vi "test5-AsyncMessageWithReply.vi"(8 "error in (no error)":errorcluster, 11 "TestCase in":refnum<class "testcase-CSMMessage.lvclass">) -> (0 "error out":errorcluster, 3 "TestCase out":refnum<class "testcase-CSMMessage.lvclass">)   [LabVIEW 2017, in "testcase-CSMMessage.lvclass"]
uses:
  testcase-CSMMessage.lvclass
  7412589e-de49-4983-aece-358686b48526.vi
  src/user.lib/_NEVSTOP/Communicable State Machine(CSM)/AdvanceAPI/CSM - Make String Arguments Safe.vi
  src/user.lib/_NEVSTOP/Communicable State Machine(CSM)/AdvanceAPI/CSM - Keywords.vi
  <vilib>/addons/_JKI Toolkits/VI Tester/TestCase.llb/TestCase.lvclass
  src/user.lib/_NEVSTOP/Communicable State Machine(CSM)/Communicable State Machine.lvlib
  C:/Program Files (x86)/National Instruments/LabVIEW 2017/vi.lib/addons/_JKI Toolkits/VI Tester/TestCase.llb/TestCase.lvclass
panel:
  out "Loop count":i32
  out "debug message":string
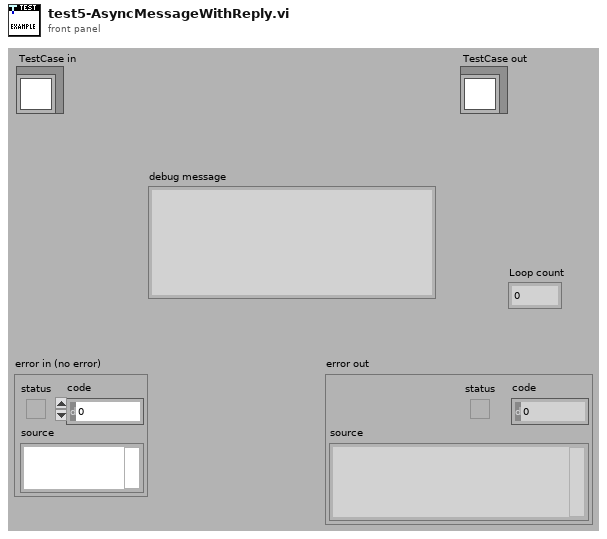
[diagram p1: front panel]
types:
  T1 = cluster{"Arguments":string, "Response":string, "error":errorcluster}
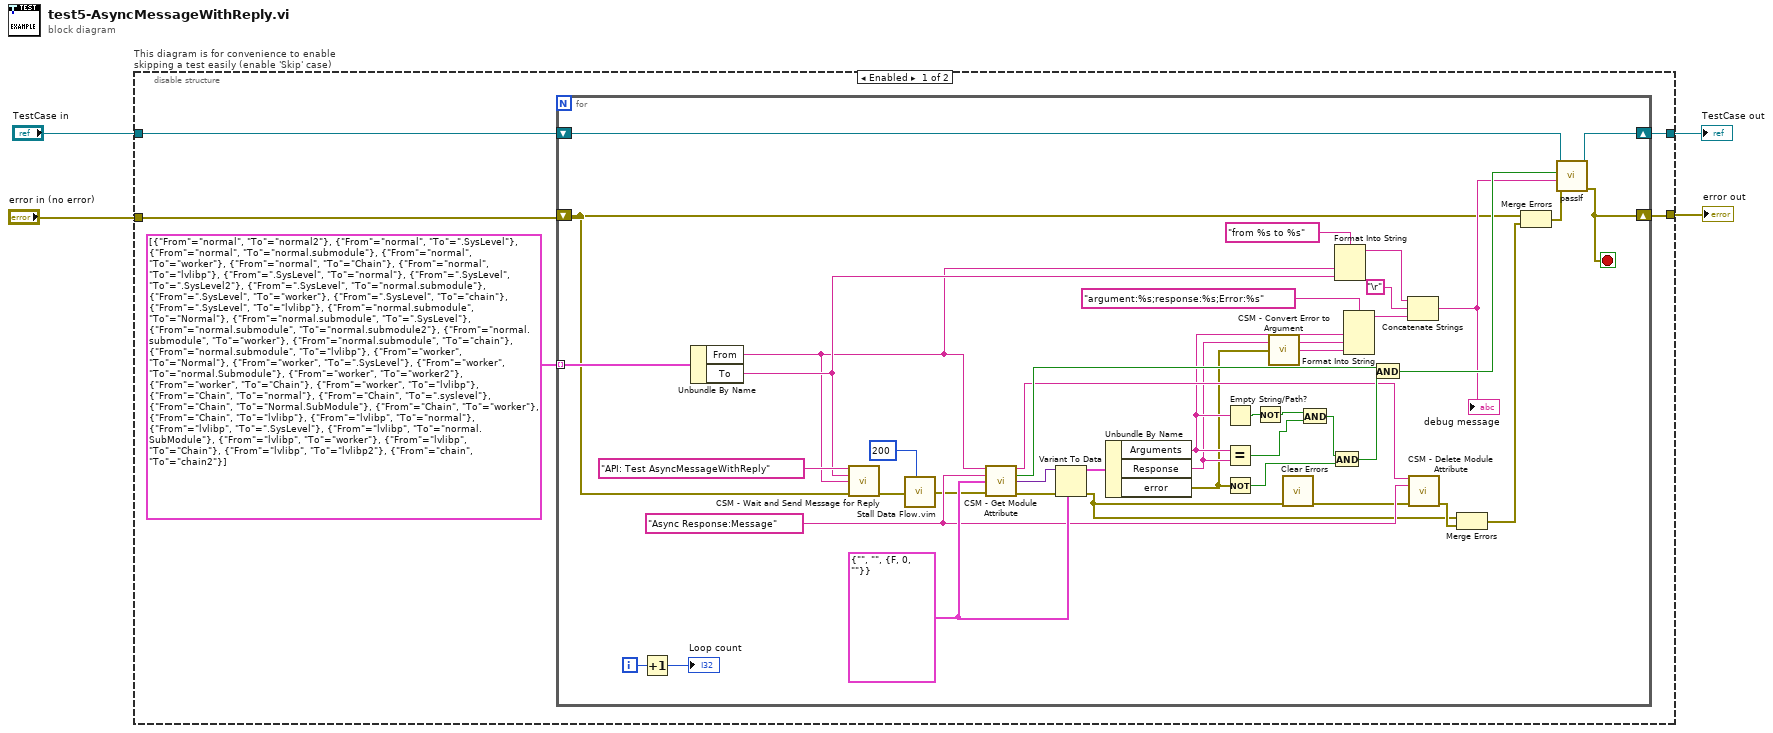
[diagram p0: block diagram]
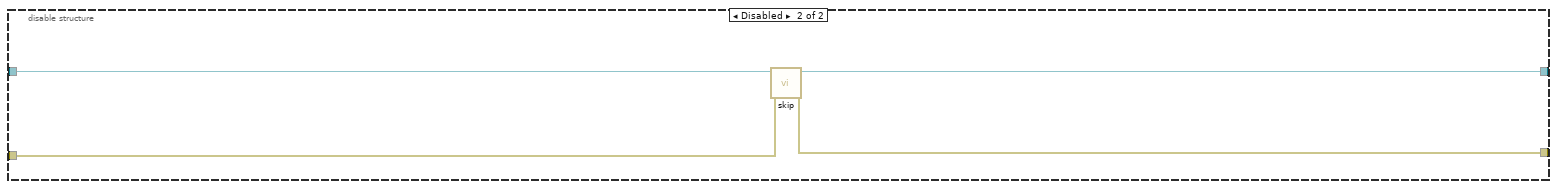
[diagram p2: hidden frame]
diagram:
  n1 = disable-structure "This diagram is for convenience to enable skipping a test easily (enable 'Skip' case)" shown="Enabled" {
    disable-tunnel: "TestCase in" -> [w9 w55]
    disable-tunnel: [w8 w53] -> w1
    disable-tunnel: [w5 w54] -> w3
    disable-tunnel: "error in (no error)" -> [w7 w52]
    frame Enabled {
      n2 = for {
        tunnel: cluster{"From":string, "To":string}[] [{"From"="normal", "To"="normal2"}, {"From"="normal", "To"=".SysLevel"}, {"From"="normal", "To"="normal.submodule"}, {"From"="normal", "To"="worker"}, {"From"="normal", "To"="Chain"}, {"From"="normal", "To"="lvlibp"}, {"From"=".SysLevel", "To"="normal"}, {"From"=".SysLevel", "To"=".SysLevel2"}, {"From"=".SysLevel", "To"="normal.submodule"}, {"From"=".SysLevel", "To"="worker"}, {"From"=".SysLevel", "To"="chain"}, {"From"=".SysLevel", "To"="lvlibp"}, {"From"="normal.submodule", "To"="Normal"}, {"From"="normal.submodule", "To"=".SysLevel"}, {"From"="normal.submodule", "To"="normal.submodule2"}, {"From"="normal.submodule", "To"="worker"}, {"From"="normal.submodule", "To"="chain"}, {"From"="normal.submodule", "To"="lvlibp"}, {"From"="worker", "To"="Normal"}, {"From"="worker", "To"=".SysLevel"}, {"From"="worker", "To"="normal.Submodule"}, {"From"="worker", "To"="worker2"}, {"From"="worker", "To"="Chain"}, {"From"="worker", "To"="lvlibp"}, {"From"="Chain", "To"="normal"}, {"From"="Chain", "To"=".syslevel"}, {"From"="Chain", "To"="Normal.SubModule"}, {"From"="Chain", "To"="worker"}, {"From"="Chain", "To"="lvlibp"}, {"From"="lvlibp", "To"="normal"}, {"From"="lvlibp", "To"=".SysLevel"}, {"From"="lvlibp", "To"="normal.SubModule"}, {"From"="lvlibp", "To"="worker"}, {"From"="lvlibp", "To"="Chain"}, {"From"="lvlibp", "To"="lvlibp2"}, {"From"="chain", "To"="chain2"}] -> [w40] mode=indexing
        shift-right: [w50] -> w8
        shift-left: w9 -> [w51]
        shift-right: [w21] -> w5
        shift-left: w7 -> [w14]
        i -> [w16]
        stop <- w21 stop-if-true
        w47 = T1 {"Arguments"="", "Response"="", "error"={"status"=FALSE, "code"=0, "source"=""}}
        w36 = "Async Response:Message" ("State")
        n3 = Increment(x=w16) -> (x+1=→"Loop count":i32)
        n4 = Unbundle By Name(w40) -> ("From"=w20:string, "To"=w39:string)
        n5 = call "CSM - Wait and Send Message for Reply.vi"("State"="API: Test AsyncMessageWithReply", "Arguments (\"\")"=w39, "Target Module"=w20, "Error In (No Error)"=w14) -> ("error out"=w18:errorcluster)  [unwired: 8 in, 3 out]
        n6 = call "Stall Data Flow.vim"("value in"=w18, "milliseconds to wait"=u32 200) -> ("value out"=w19:errorcluster)  [unwired: 1 out]
        n7 = call "CSM - Get Module Attribute.vi"("CSM Name"=w20, "Attribute"=w36, "Default Value (Empty Variant)"=w47, "Error In"=w19) -> ("CSM Name (Dup)"=w37:string, "Found"=w43:bool, "Value"=w46:variant, "error out"=w48:errorcluster)  [unwired: 7 in, 1 out]
        n8 = Variant To Data(error in=w48, type=w47, Variant=w46) -> (data=w45:T1, error out=w12:errorcluster)
        n9 = Unbundle By Name(w45) -> ("Arguments"=w31:string, "Response"=w30:string, "error"=w28:errorcluster)
        n10 = Empty String/Path?(string/path=w31) -> (empty?=w35:bool)
        n11 = Equal?(x=w31, y=w30) -> (x = y?=w33:bool)
        n12 = Not(x=w28) -> (.not. x?=w44:bool)
        n13 = Not(x=w35) -> (.not. x?=w34:bool)
        n14 = call "CSM - Convert Error to Argument.vi"("Error"=w28) -> ("Argument"=w29:string)  [unwired: 4 in]
        n15 = call <vilib>:"Clear Errors.vi"("error in (no error)"=w12) -> ("error out"=w22:errorcluster)  [unwired: 5 in, 1 out]
        n16 = And(x=w34, y=w33) -> (x .and. y?=w32:bool)
        n17 = And(x=w32, y=w44) -> (x .and. y?=w42:bool)
        n18 = Format Into String(format string="from %s to %s", w20, w39) -> (resulting string=w24:string)  [unwired: 2 in, 1 out]
        n19 = Format Into String(format string="argument:%s;response:%s;Error:%s", w31, w30, w29) -> (resulting string=w27:string)  [unwired: 2 in, 1 out]
        n20 = And(x=w43, y=w42) -> (x .and. y?=w41:bool)
        n21 = Concatenate Strings(w24, "\r", w27) -> (w25:string)
        "debug message" <- w25
        n22 = call "CSM - Delete Module Attribute.vi"("CSM Name"=w37, "Attribute"=w36, "Error In"=w22) -> ("error out"=w13:errorcluster)  [unwired: 9 in, 3 out]
        n23 = Merge Errors(w12, w13) -> (w10:errorcluster)
        n24 = Merge Errors(w14, w10) -> (w11:errorcluster)
        n25 = call-dynamic "passIf.vi"("error in (no error)"=w11, "message (\"\")"=w25, "pass"=w41, "TestCase in"=w51) -> ("error out"=w21:errorcluster, "TestCase out"=w50:refnum<class "testcase-CSMMessage.lvclass">)  [unwired: 6 in]
      }
    }
    frame Disabled {
      # "skip test result while test is under development"
      n26 = call <vilib>:"skip.vi"("error in (no error)"=w52, "TestCase in"=w55) -> ("error out"=w54:errorcluster, "TestCase out"=w53:refnum<class "testcase-CSMMessage.lvclass">)  [unwired: 8 in]
    }
  }
  "error out" <- w3
  "TestCase out" <- w1
